vi "Get Test.vi"(8 "error in (no error)":errorcluster, 10 "Unique ID":string, 11 "Test Executive in":refnum<class "Test Executive.lvclass">) -> (0 "error out":errorcluster, 1 "Found?":bool, 2 "Test":refnum<class "Executioner.lvclass">, 3 "Test Executive out":refnum<class "Test Executive.lvclass">)   [LabVIEW 2017, in "Test Executive.lvlib" / "Test Executive.lvclass"]
uses:
  <vilib>/gpm_packages/@cs/test-executive/Source/Test Executive/TestExecutive/Test Executive.lvclass
  <vilib>/gpm_packages/@cs/test-executive/Source/Test Executive/Executioner/Executioner.lvclass
  <vilib>/gpm_packages/@cs/test-executive/Source/Test Executive/TestExecutive/Test Executive.lvclass/Test Executive.ctl
  <vilib>/gpm_packages/@cs/linked-list/Source/Linked List/Linked List Ref/Linked List Ref.lvclass
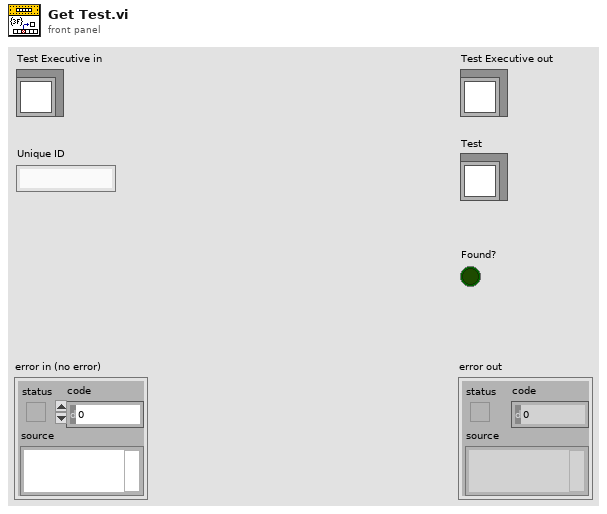
[diagram p1: front panel]
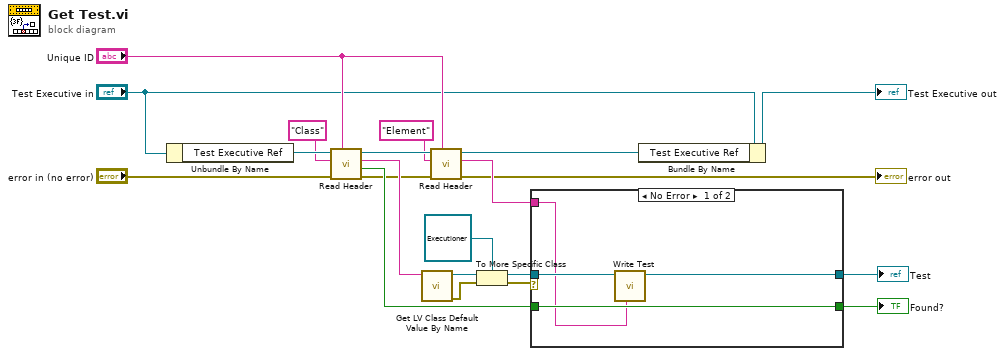
[diagram p0: block diagram]
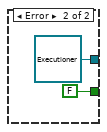
[diagram p2: hidden frame]
diagram:
  n1 = Unbundle By Name("Test Executive in") -> ("Test Executive Ref"=w21:refnum<data-value>)
  n2 = call <vilib>:"Read Header.vi"("Linked List ID"="Unique ID", "error in (no error)"="error in (no error)", "Header Name"="Class", "Linked List Ref"=w21) -> ("error out"=w9:errorcluster, "found"=w13:bool, "Header Value"=w19:string, "Linked List Ref out"=w10:refnum<data-value>)  [unwired: 4 in]
  n3 = call <vilib>:"Get LV Class Default Value By Name.vi"("class name"=w19) -> ("error out"=w16:errorcluster, "object"=w18:refnum<class>)  [unwired: 9 in]
  n4 = call <vilib>:"Read Header.vi"("Linked List ID"="Unique ID", "error in (no error)"=w9, "Header Name"="Element", "Linked List Ref"=w10) -> ("error out"=→"error out":errorcluster, "Header Value"=w6:string, "Linked List Ref out"=w2:refnum<data-value>)  [unwired: 4 in, 1 out]
  n5 = To More Specific Class(target class=refnum<class "Executioner.lvclass"> refnum ("Test Executive.lvlib:Executioner.lvclass"), reference=w18, error in=w16) -> (specific class reference=w14:refnum<class "Executioner.lvclass">, error out=w15:errorcluster)
  n6 = case shown="No Error" w15 {
    tunnel: w14 -> [w24 _]
    tunnel: w13 -> [w25 _]
    tunnel: [w25 FALSE ("found")] -> w12
    tunnel: w6 -> [w23 _]
    tunnel: [w22 refnum<class "Executioner.lvclass"> refnum ("Executioner out")] -> w5
    frame No Error {
      n7 = call <vilib>:"Write Test.vi"("Test"=w23, "Executioner in"=w24) -> ("Executioner out"=w22:refnum<class "Executioner.lvclass">)  [unwired: 9 in]
    }
    frame Error {
    }
  }
  "Found?" <- w12
  "Test" <- w5
  n8 = Bundle By Name(cluster="Test Executive in", "Test Executive Ref"=w2) -> (→"Test Executive out":refnum<class "Test Executive.lvclass">)
